vi "Gen_Apply Config.vi"(8 "错误输入":errorcluster caption="错误输入（无错误）", 11 "Cards in":T1[](array[typedef])) -> (0 "错误输出":errorcluster, 2 "Success?":bool, 3 "Cards out":T1[](array[typedef]))   [LabVIEW 2016]
uses:
  DAQ-Config/Controls/PSCHN_Channel Para.ctl
  DAQ-Config/Controls/PSCHN_Card Para.ctl
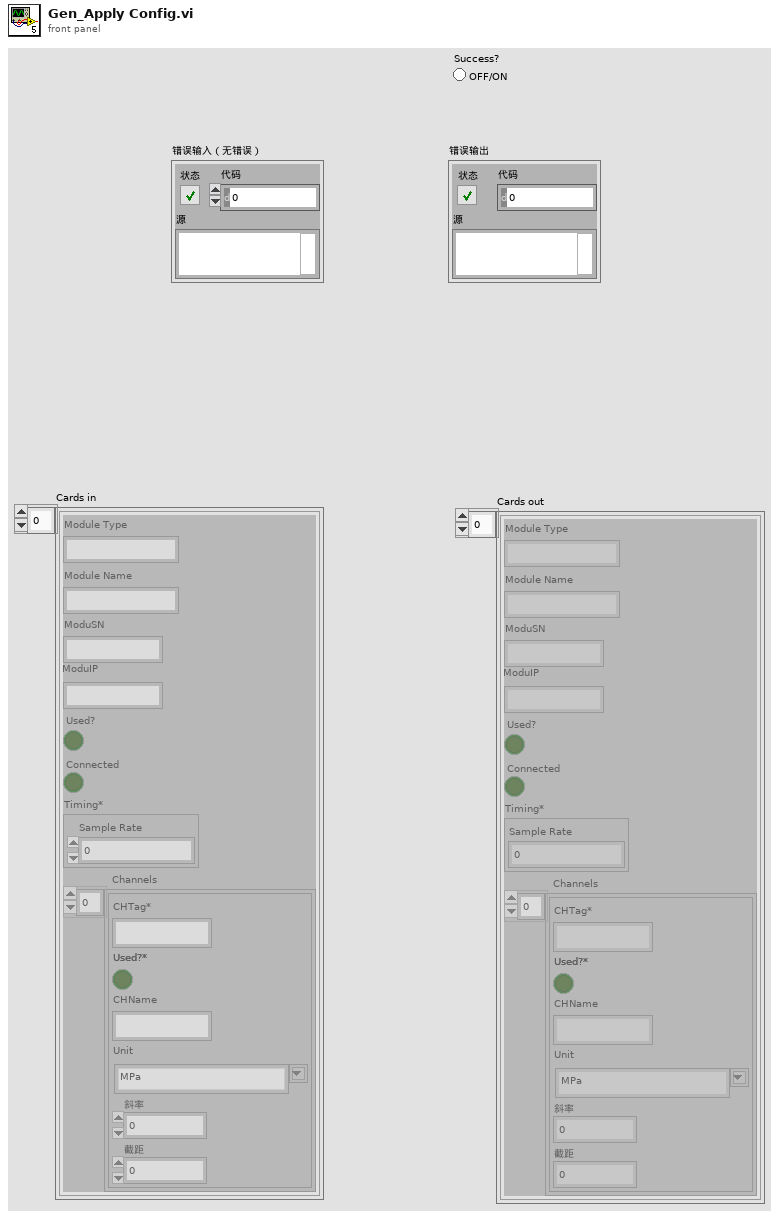
[diagram p1: front panel]
types:
  T1 = typedef "PSCHN_Card Para.ctl" = cluster{"Module Type":string, "Module Name":string, "ModuSN":string, "ModuIP":string, "Used?":bool, "Connected":bool, "Timing*":cluster{"Sample Rate":dbl}, "Channels":T2[]}
  T2 = typedef "PSCHN_Channel Para.ctl" = cluster{"CHTag*":string, "Used?*":bool, "CHName":string, "Unit":string, "斜率":dbl, "截距":dbl}
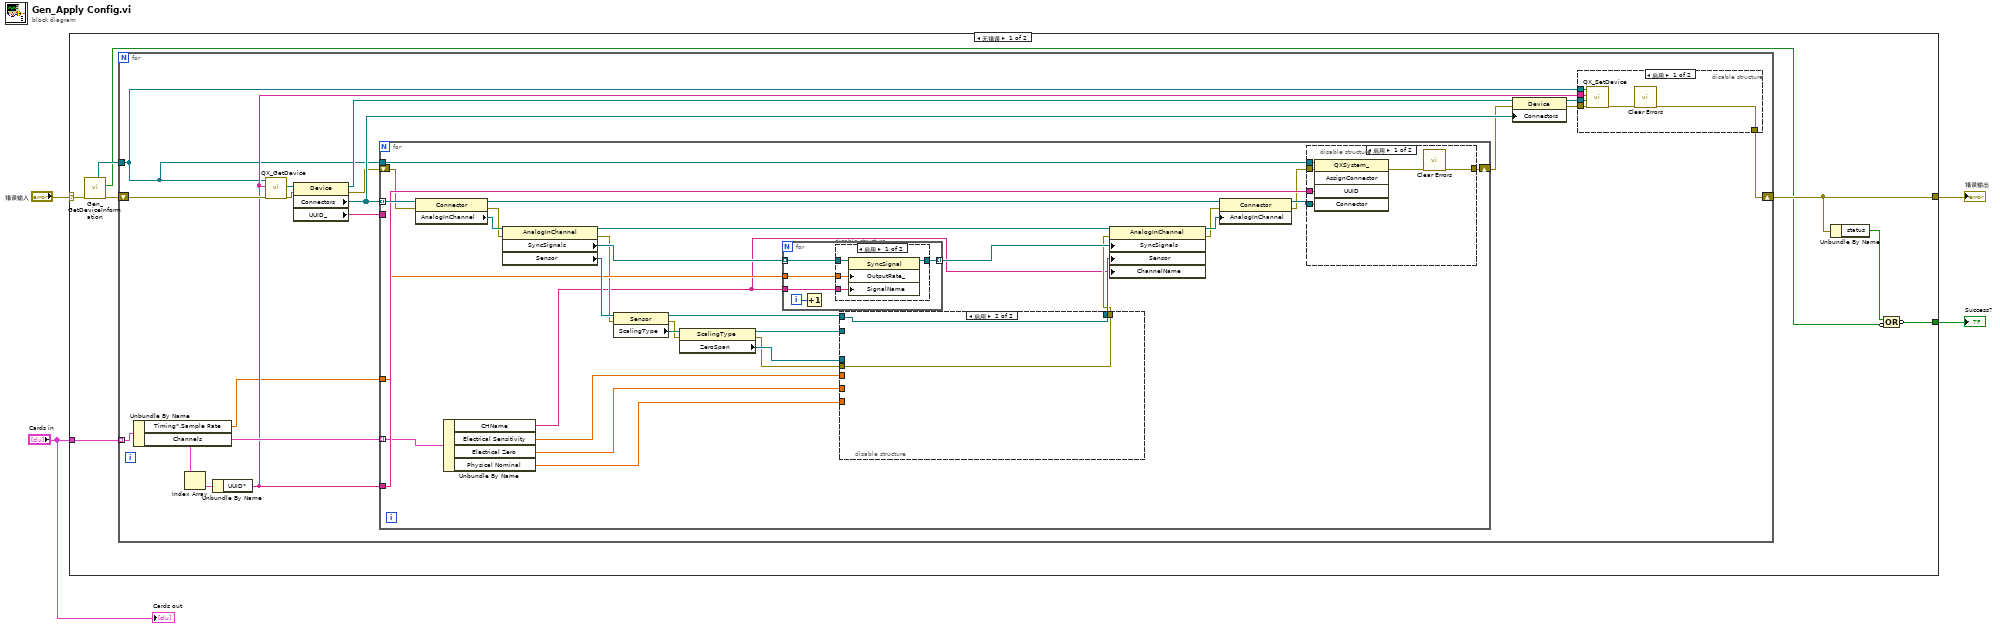
[diagram p0: block diagram]
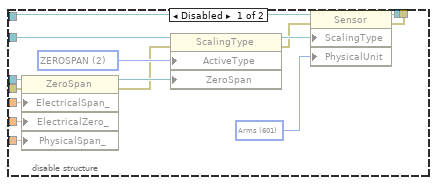
[diagram p4: hidden frame]
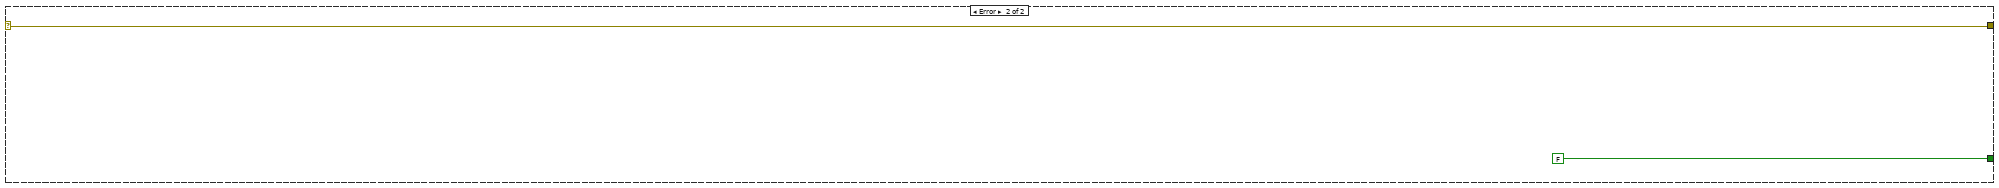
[diagram p6: hidden frame]
diagram:
  n1 = case shown="无错误" "错误输入" {
    selector: "错误输入" -> [w12 w103]
    tunnel: [w8 w103] -> w4
    tunnel: [w5 FALSE] -> w2
    tunnel: "Cards in" -> [w11 _]
    frame No Error {
      n2 = call "Gen_GetDeviceInformation.vi"("error"=w12) -> ("错误输出"=w10:errorcluster, "Succeed"=w6:bool, "QXSystem reference"=w9:refnum<k24>)  [unwired: 6 in, 2 out]
      n3 = for {
        tunnel: w11 -> [w27] mode=indexing
        shift-right: [w19] -> w8
        shift-left: w10 -> [w28]
        tunnel: w9 -> [w14]
        n4 = Unbundle By Name(w27) -> ("Timing*.Sample Rate"=w15:dbl, "Channels"=w25:T2[])
        n5 = Index Array(array=w25) -> (element=w26:T2)  [unwired: 1 in]
        n6 = Unbundle By Name(w26) -> ("UUID*"=w21:string)
        n7 = call <userlib>:"QX_GetDevice.vi"("error in"=w28, "UUID"=w21, "QXSystem reference"=w14) -> ("error out"=w17:errorcluster, "Device reference"=w29:refnum<k24>)  [unwired: 6 in, 1 out]
        n8 = property on="属性节点" class="Device"(reference=w29, error in=w17) -> (reference out=w23:refnum<k24>, error out=w16:errorcluster, "Connectors"=w22:refnum<k24>[], "UUID_"=w13:string)
        n9 = for {
          tunnel: w25 -> [w47] mode=indexing
          tunnel: w22 -> [w64] mode=indexing
          tunnel: w14 -> [w52]
          tunnel: w21 -> [w54]
          shift-right: [w37] -> w18
          shift-left: w16 -> [w51]
          tunnel: w15 -> [w43]
          tunnel: w13 -> [_]
          n10 = property on="属性节点" class="Connector"(reference=w64, error in=w51) -> (reference out=w55:refnum<k24>, error out=w50:errorcluster, "AnalogInChannel"=w67:refnum<k24>)
          n11 = Unbundle By Name(w47) -> ("CHName"=w38:string, "Electrical Sensitivity"=w46:dbl, "Electrical Zero"=w45:dbl, "Physical Nominal"=w44:dbl)
          n12 = property on="属性节点" class="AnalogInChannel"(reference=w67, error in=w50) -> (reference out=w57:refnum<k24>, error out=w42:errorcluster, "SyncSignals"=w60:refnum<k24>[], "Sensor"=w66:refnum<k24>)
          n13 = property class="Sensor"(reference=w66, error in=w42) -> (reference out=w61:refnum<k24>, error out=w41:errorcluster, "ScalingType"=w65:refnum<k24>)
          n14 = property class="ScalingType"(reference=w65, error in=w41) -> (reference out=w62:refnum<k24>, error out=w40:errorcluster, "ZeroSpan"=w63:refnum<k24>)
          n15 = for {
            tunnel: w60 -> [w96] mode=indexing
            tunnel: [w95] -> w59 mode=indexing
            tunnel: w43 -> [w92]
            tunnel: w38 -> [w94]
            i -> [w93]
            n16 = Increment(x=w93) -> ()  [unwired: 1 out]
            n17 = disable-structure shown="启用" {
              disable-tunnel: w96 -> [w100 w101]
              disable-tunnel: [w99 w101] -> w95
              disable-tunnel: w94 -> [w98 _]
              disable-tunnel: w92 -> [w97 _]
              frame Enabled {
                n18 = property on="属性节点" class="SyncSignal"(reference=w100, "OutputRate_"=w97, "SignalName"=w98) -> (reference out=w99:refnum<k24>)  [unwired: 1 in, 1 out]
              }
              frame Disabled {
              }
            }
          }
          n19 = disable-structure shown="启用" {
            disable-tunnel: w63 -> [w83 _]
            disable-tunnel: w62 -> [w82 _]
            disable-tunnel: w61 -> [w81 w91]
            disable-tunnel: [w80 w91] -> w58
            disable-tunnel: w46 -> [w79 _]
            disable-tunnel: w45 -> [w78 _]
            disable-tunnel: w44 -> [w77 _]
            disable-tunnel: w40 -> [w76 w90]
            disable-tunnel: [w75 w90] -> w39
            frame Disabled {
              w89 = 601 items=["none"=0, "rad"=100, "radian"=101, "o"=102, "percento"=103, "m"=300, "micrometer, um"=301, "mm"=302, "cm"=303, "dm"=304, "km"=305, "inch"=306, "feet"=307, "yard"=308, "mile"=309, "kg"=400, "g"=401, "t"=402, "kt"=403, "tons"=404, "lbs"=405, "s"=500, "ms"=501, "microsecond, us"=502, "min"=503, "h"=504, "days"=505, "A"=600, "Arms"=601, "mA"=602, "uA"=603, "mArms"=604, "uArms"=605, "K"=700, "oC"=701, "oF"=702, "oRank"=703, "oR"=704, "V_V"=1000, "mV_V"=1001, "uV_V"=1002, "V"=1100, "mV"=1101, "microvolt, uV"=1102, "Vrms"=1103, "mVrms"=1104, "microvoltrms, uVrms"=1105, "Ohm"=1200, "kOhm"=1201, "MOhm_"=1202, "mOhm"=1203, "H_"=1300, "mH"=1301, "uH, microH"=1302, "nH"=1303, "F"=1400, "mF"=1401, "microF, uF"=1402, "nF"=1403, "pF"=1404, "C"=1500, "nC"=1501, "pC"=1502, "Hz"=1600, "kHz"=1601, "MHz"=1602, "One_s"=1603, "mHz_"=1604, "radian_s"=1700, "U_min"=1701, "rpm"=1702, "One_min"=1703, "W"=1800, "mW"=1801, "kW"=1802, "MW_"=1803, "GW"=1804, "N"=1900, "kN"=1901, "MN"=1902, "kp"=1903, "kgf"=1904, "lb"=1905, "GN"=1906, "Pa"=2000, "bar"=2001, "mbar"=2002, "kbar"=2003, "pas"=2004, "hPa"=2005, "kPa"=2006, "psi"=2007, "N_mm2"=2008, "N_m2"=2009, "N_cm2"=2010, "MPa"=2011, "GPa"=2012, "J"=2100, "Nm"=2101, "kNm"=2102, "MNm"=2103, "ftlb"=2104, "inlb"=2105, "GNm"=2106, "Nm_radian"=2107, "ozin"=2108, "Nm_"=2200, "m_m"=2300, "um_m, microstrain"=2301, "strain"=2302, "mm_m"=2303, "m_s"=2400, "km_h"=2401, "mph"=2402, "fps"=2403, "m_h"=2404, "m_s2"=2500, "ga"=2501, "mm_s2"=2502, "kg_m3"=2700, "g_l"=2701, "m3_s"=2800, "l_min"=2801, "m3_h"=2802, "gpm"=2803, "cfm"=2804, "l_h"=2805, "l_s"=2806, "percent"=2900, "promill"=2901, "ppm"=2902, "percent_oC"=3000, "promill_oC"=3001, "ppm_oC"=3002, "Imp"=3100, "kImp"=3101, "percent_decade"=5001, "dB"=5002, "l_l"=5003, "m3_m3"=5004, "m3"=5005, "mm2"=5006, "kg_s"=5007, "mole_l"=5008, "mole_m3"=5009, "N_m"=5010, "RH"=5011, "V__m_s2"=5012, "V_C"=5013, "V_N"=5014, "V_PA"=5015, "W_oC"=5016, "UserDefined"=100000, "UNKNOWN"=-1] ("PhysicalUnit")
              w88 = 2 items=["OFF"=0, "INTERNAL"=1, "ZEROSPAN"=2, "POLYNOM"=3, "LINTABLE"=4, "GAIN"=5, "STRAINGAGE"=6, "UNKNOWN"=-1] ("ActiveType")
              n20 = property class="ZeroSpan"(reference=w83, error in=w76, "ElectricalSpan_"=w79, "ElectricalZero_"=w78, "PhysicalSpan_"=w77) -> (reference out=w86:refnum<k24>, error out=w85:errorcluster)
              n21 = property class="ScalingType"(reference=w82, error in=w85, "ActiveType"=w88, "ZeroSpan"=w86) -> (reference out=w87:refnum<k24>, error out=w84:errorcluster)
              n22 = property class="Sensor"(reference=w81, error in=w84, "ScalingType"=w87, "PhysicalUnit"=w89) -> (reference out=w80:refnum<k24>, error out=w75:errorcluster)
            }
            frame Enabled {
            }
          }
          n23 = property on="属性节点" class="AnalogInChannel"(reference=w57, error in=w39, "SyncSignals"=w59, "Sensor"=w58, "ChannelName"=w38) -> (reference out=w56:refnum<k24>, error out=w49:errorcluster)
          n24 = property on="属性节点" class="Connector"(reference=w55, error in=w49, "AnalogInChannel"=w56) -> (reference out=w53:refnum<k24>, error out=w48:errorcluster)
          n25 = disable-structure shown="启用" {
            disable-tunnel: w54 -> [w73 _]
            disable-tunnel: w53 -> [w72 _]
            disable-tunnel: w52 -> [w71 _]
            disable-tunnel: w48 -> [w70 w74]
            disable-tunnel: [w68 w74] -> w37
            frame Enabled {
              n26 = invoke class="QXSystem_" method="AssignConnector"(reference=w71, error in=w70, "UUID"=w73, "Connector"=w72) -> (error out=w69:errorcluster)  [unwired: 1 in, 4 out]
              n27 = call <vilib>:"Clear Errors.vi"("error in (no error)"=w69) -> ("error out"=w68:errorcluster)  [unwired: 5 in, 1 out]
            }
            frame Disabled {
            }
          }
        }
        n28 = property on="属性节点" class="Device"(reference=w23, error in=w18, "Connectors"=w22) -> (reference out=w24:refnum<k24>, error out=w20:errorcluster)
        n29 = disable-structure shown="启用" {
          disable-tunnel: w24 -> [w35 _]
          disable-tunnel: w14 -> [w34 _]
          disable-tunnel: w21 -> [w33 _]
          disable-tunnel: w20 -> [w32 w36]
          disable-tunnel: [w30 w36] -> w19
          frame Enabled {
            n30 = call <userlib>:"QX_SetDevice.vi"("error in"=w32, "Device reference"=w35, "UUID"=w33, "QXSystem reference"=w34) -> ("error out"=w31:errorcluster)  [unwired: 6 in, 1 out]
            n31 = call <vilib>:"Clear Errors.vi"("error in (no error)"=w31) -> ("error out"=w30:errorcluster)  [unwired: 5 in, 1 out]
          }
          frame Disabled {
          }
        }
      }
      n32 = Unbundle By Name(w8) -> ("status"=w7:bool)
      n33 = Compound Arithmetic op=OR(w7, invert w6) -> (invert w5:bool)
    }
    frame Error {
    }
  }
  "错误输出" <- w4
  "Success?" <- w2
  "Cards out" <- "Cards in"
